vi "Create Channels.vi"(8 "error in (no error)":errorcluster, 10 "RSI Module in":refnum<class "9207.lvclass">, 11 "Parent Ref in":T1 format="%.0x") -> (0 "error out":errorcluster, 2 "RSI Module out":refnum<class "9207.lvclass">, 3 "Parent Ref out":T1 format="%.0x")   [LabVIEW 2020, in "Modules.lvlib" / "9207.lvclass"]
uses:
  9207.lvclass
  C:/Users/nitest/Desktop/Git 2020/niveristand-scan-engine-module-libraries/Source/RSI Module/RSI Module.lvclass
  <vilib>/NI VeriStand/Custom Device API/Custom Device Item Ref.ctl
  <vilib>/NI VeriStand/Custom Device API/Custom Device Channel.ctl
  <vilib>/NI VeriStand/Custom Device API/Custom Device Channel Type.ctl
  RSI Module/Class Property Strings.vi
  RSI Module/Channel GUIDs.vi
  RSI Module/RSI Module.lvclass
  <vilib>/NI VeriStand/Custom Device API/Custom Device API.lvlib
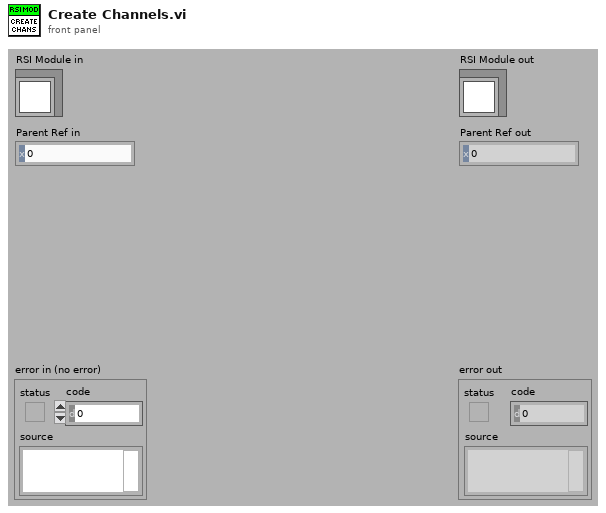
[diagram p1: front panel]
types:
  T1 = typedef "Custom Device API.lvlib/Custom Device Item Ref.ctl" = u64
  T2 = typedef "Custom Device API.lvlib/Custom Device Channel.ctl" = cluster{"Type":T3, "Units":string, "Default Value":dbl, "Faultable":bool, "Scalable":bool}
  T3 = typedef "Custom Device API.lvlib/Custom Device Channel Type.ctl" = enum16{"Input", "Output"}
  T4 = typedef "Modules.lvlib/RSI Module.lvclass/Module Models.ctl" = enum16{"Empty", "NI 9201", "NI 9203", "NI 9205", "NI 9206", "NI 9207", "NI 9208", "NI 9209", "NI 9210", "NI 9211", "NI 9212", "NI 9213", "NI 9214", "NI 9215", "NI 9216", "NI 9217", "NI 9219", "NI 9220", "NI 9221", "NI 9222", "NI 9223", "NI 9224", "NI 9225", "NI 9226", "NI 9227", "NI 9228", "NI 9229", "NI 9233", "NI 9234", "NI 9235", "NI 9236", "NI 9237", "NI 9239", "NI 9242", "NI 9244", "NI 9253", "NI 9263", "NI 9264", "NI 9265", "NI 9266", "NI 9269", "NI 9344", "NI 9350", "NI 9375", "NI 9401", "NI 9402", "NI 9403", "NI 9411", "NI 9421", "NI 9422", "NI 9423", "NI 9425", "NI 9426", "NI 9435", "NI 9436", "NI 9437", "NI 9472", "NI 9474", "NI 9475", "NI 9476", "NI 9477", "NI 9478", "NI 9481", "NI 9482", "NI 9485"}
  T5 = typedef "Modules.lvlib/RSI Module.lvclass/Channels.ctl" = cluster{"# Input Channels":i32, "# Output Channels":i32, "Channel Type":T6, "Units":string}
  T6 = typedef "Modules.lvlib/RSI Module.lvclass/Channel Type.ctl" = enum16{"Analog", "Digital"}
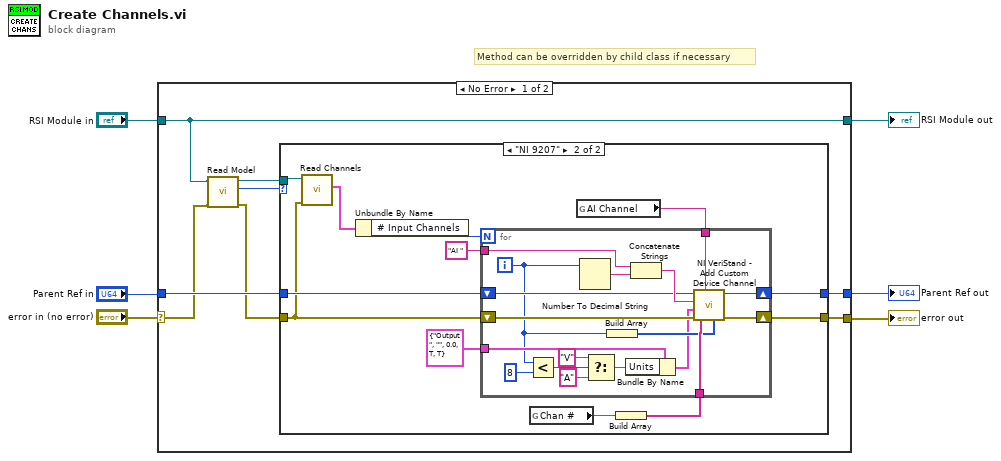
[diagram p0: block diagram]
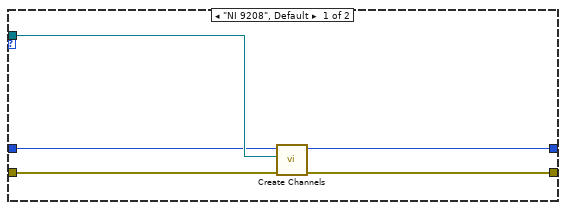
[diagram p2: hidden frame]
diagram:
  # "Method can be overridden by child class if necessary"
  n1 = case shown="No Error" "error in (no error)" {
    selector: "error in (no error)" -> [w11 w52]
    tunnel: [w13 w52] -> w5
    tunnel: [w9 w51] -> w3
    tunnel: "RSI Module in" -> [w9 w51]
    tunnel: "Parent Ref in" -> [w14 w50]
    tunnel: [w12 w50] -> w1
    frame No Error {
      n2 = call "Read Model.vi"("error in (no error)"=w11, "RSI Module in"=w9) -> ("error out"=w10:errorcluster, "Model"=w8:T4, "RSI Module out"=w7:refnum<class "9207.lvclass">)  [unwired: 7 in]
      n3 = case shown="\"NI 9207\"" w8 {
        tunnel: w14 -> [w18 w31]
        tunnel: [w15 w28] -> w13
        tunnel: [w16 w27] -> w12
        tunnel: w10 -> [w17 w25]
        tunnel: w7 -> [w19 w24]
        frame "NI 9208", Default {
          n4 = call-parent "Create Channels.vi"("error in (no error)"=w17, "RSI Module in"=w19, "Parent Ref in"=w18) -> ("error out"=w15:errorcluster, "Parent Ref out"=w16:T1)  [unwired: 6 in, 1 out]
        }
        frame "NI 9207" {
          n5 = call "Read Channels.vi"("error in (no error)"=w25, "RSI Module in"=w24) -> ("Channels"=w23:T5)  [unwired: 7 in, 2 out]
          n6 = Unbundle By Name(w23) -> ("# Input Channels"=w22:i32)
          n7 = global read "Class Property Strings.vi" "Chan #"() -> (w30:string)
          n8 = global read "Channel GUIDs.vi" "AI Channel"() -> (w21:string)
          n9 = Build Array(w30) -> (w29:string[])
          n10 = for {
            N: w22 -> [_]
            tunnel: "AI " ("Channel Name") -> [w47]
            tunnel: w29 -> [w44]
            shift-right: [w42] -> w28
            shift-left: w25 -> [w48]
            shift-right: [w41] -> w27
            shift-left: w31 -> [w45]
            tunnel: w21 -> [w40]
            tunnel: T2 {"Type"=enum."Output", "Units"="", "Default Value"=0.0, "Faultable"=TRUE, "Scalable"=TRUE} ("Channel") -> [w39]
            i -> [w38]
            n11 = Less?(x=w38, y=8) -> (x < y?=w36:bool)
            n12 = Number To Decimal String(number=w38) -> (decimal integer string=w49:string)  [unwired: 1 in]
            n13 = Select(t="V" ("Units"), s=w36, f="A" ("Units")) -> (s? t:f=w33:string)
            n14 = Build Array(w38) -> (w43:i32[])
            n15 = Bundle By Name(cluster=w39, "Units"=w33) -> (w32:T2)
            n16 = Concatenate Strings(w47, w49) -> (w46:string)
            n17 = call <vilib>:"NI VeriStand - Add Custom Device Channel.vi"("Property Values"=w43, "Property names"=w44, "GUID (Default Channel)"=w40, "error in (no error)"=w48, "Channel"=w32, "Channel Name"=w46, "Parent Ref in"=w45) -> ("error out"=w42:errorcluster, "Parent Ref out"=w41:T1)  [unwired: 1 in, 2 out]
          }
        }
      }
    }
    frame Error {
    }
  }
  "error out" <- w5
  "RSI Module out" <- w3
  "Parent Ref out" <- w1
